vi "Enter_Temp_Press.vi"() -> ()   [LabVIEW 2020]
uses:
  Sub VIs/ADAM Controls/Channel_names.ctl
  Anemometry/Anemometry Sub Vis/Globals/Preference_global.vi
  Anemometry/Anemometry Sub Vis/Globals/Constants_global.vi
  Sub VIs/ADAM Controls/Module_type_ADAM.ctl
  Anemometry/Anemometry Sub Vis/Controls/Preference_Mode.ctl
  Anemometry/Anemometry Sub Vis/File/Setup_Filetype.ctl
  Anemometry/Anemometry Sub Vis/Controls/Server_Comms.ctl
  Sub VIs/ADAM Controls/Update_scan_value.ctl
  <vilib>/Utility/config.llb/NI_LVConfig.lvlib
  <vilib>/Utility/config.llb/Write Key (String).vi
  <vilib>/Utility/config.llb/Write Key (I32).vi
  Sub VIs/ADAM Controls/Function_ADAM.ctl
  Sub VIs/ADAM Controls/Channel_State.ctl
  Sub VIs/ADAM Controls/Calib_type_ADAM.ctl
  Sub VIs/ADAM Controls/Address.ctl
  Sub VIs/ADAM Controls/Ch_description_ADAM.ctl
panel:
  in  "OK":bool
  out "Ch Description Array":T1[](array[typedef]) {"Duty" format="%016b"; "D" format="%#_5g"; "C" format="%#_5g"; "B" format="%#_5g"; "A" format="%#_5g"}
  in  "mbars":dbl format="%#.1f"
  in  "Deg C":dbl format="%#.1f"
  in  "type specifier VI Refnum (for type only)":refnum<vi>
  out "Preference file":path
  in  "Server Comms":T7=enum."Server Link Healthy"
  in  "Browse for Atmos Press":bool
  in  "Browse for Temp Ch":bool
  in  "Flow Pressure (Absolute) (mbars)":string="Froude:NPL:Atmos_Press"
  in  "Flow Temperature (deg C)":string="EnFlo Tun:Inlet Heater:Av Temp"
  # "DATA SOURCE"
  # "CURRENT VALUES"
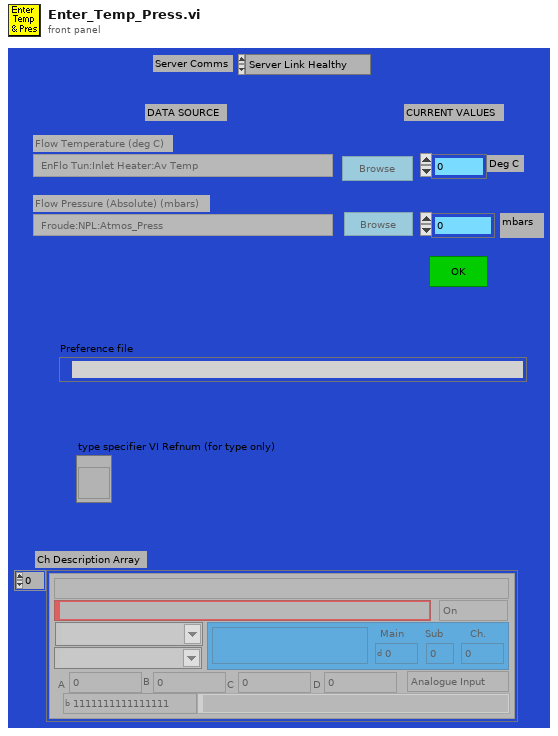
[diagram p1: front panel]
types:
  T1 = typedef "Ch_description_ADAM.ctl" = cluster{"Ch Name":string, "Type":T2, "Function":T3, "Ch State":T4, "Calibration type":T5, "A":dbl, "B":dbl, "C":dbl, "D":dbl, "Comments":string, "Address":T6, "String":string, "Duty":u16}
  T2 = typedef "Module_type_ADAM.ctl" = string
  T3 = typedef "Function_ADAM.ctl" = enum16{"Analogue Input", "Digital Input", "Event counter", "Event rate", "Analogue Output", "Digital Output", "Relay Output"}
  T4 = typedef "Channel_State.ctl" = enum16{"On", "Off", "Always On", "Always Off"}
  T5 = typedef "Calib_type_ADAM.ctl" = string
  T6 = typedef "Address.ctl" = cluster{"Main":i32, "Ch.":i32, "Sub":i32, "Port Name":string}
  T7 = typedef "Server_Comms.ctl" = enum16{"Do Not Link To Server", "Server Link Healthy"}
  T8 = typedef "Setup_Filetype.ctl" = enum16{"Measurement Setups", "Calibration Setups", "General", "Results File Plotter Setups", "Speed Calib Tweaks"}
  T9 = typedef "Channel_names.ctl" = enum16{"Active Only", "Active + Off", "All Channels"}
  T10 = enum16{"Zero or one", "One", "Zero or more", "One or more"}
  T11 = typedef "Preference_Mode.ctl" = enum16{"Load Preferences from file", "Save Preferences to file", "Load, Edit then Save"}
  T12 = typedef "Update_scan_value.ctl" = cluster{"Channel Name":string, "New Value":dbl}
  T13 = typedef "NI_LVConfig.lvlib/Config Data RefNum.ctl" = refnum<k1>
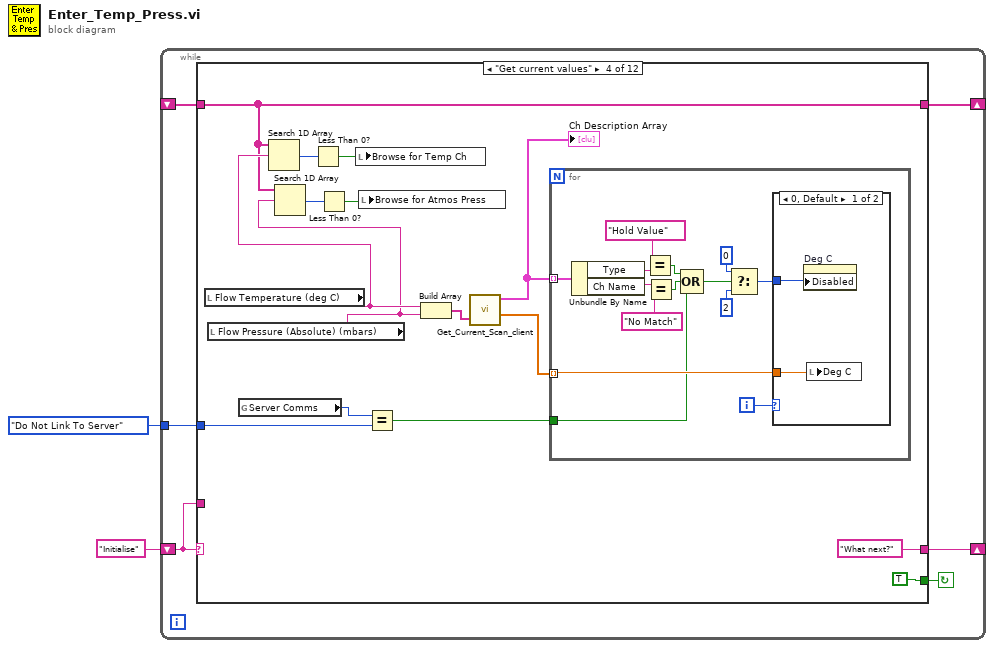
[diagram p0: block diagram]
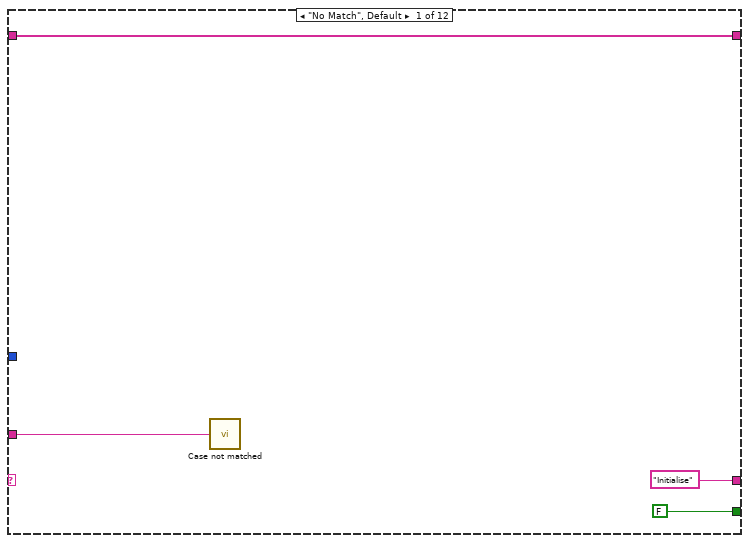
[diagram p2: hidden frame]
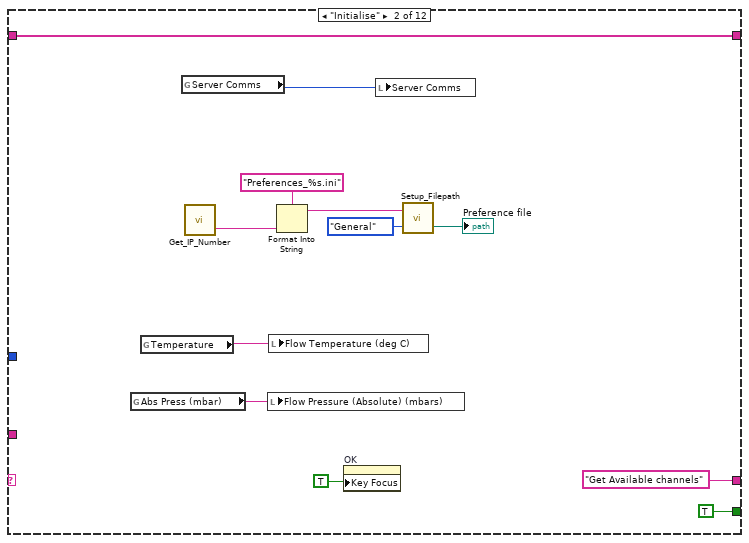
[diagram p3: hidden frame]
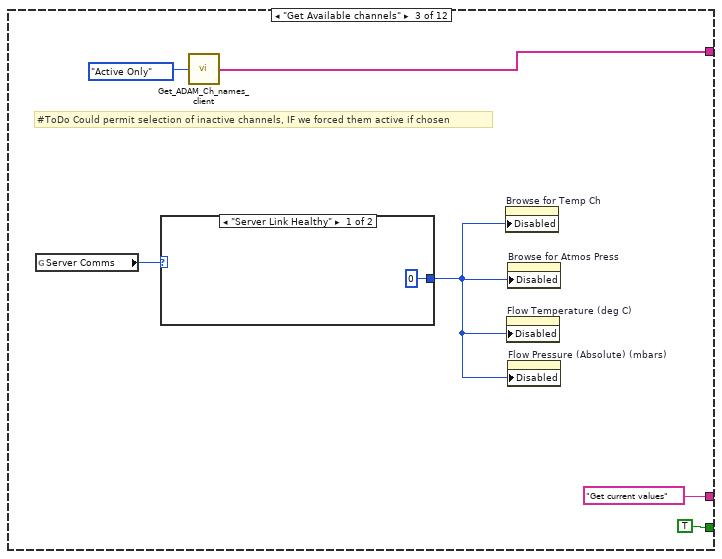
[diagram p4: hidden frame]
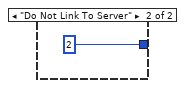
[diagram p5: hidden frame]
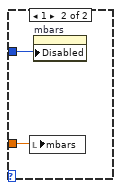
[diagram p6: hidden frame]
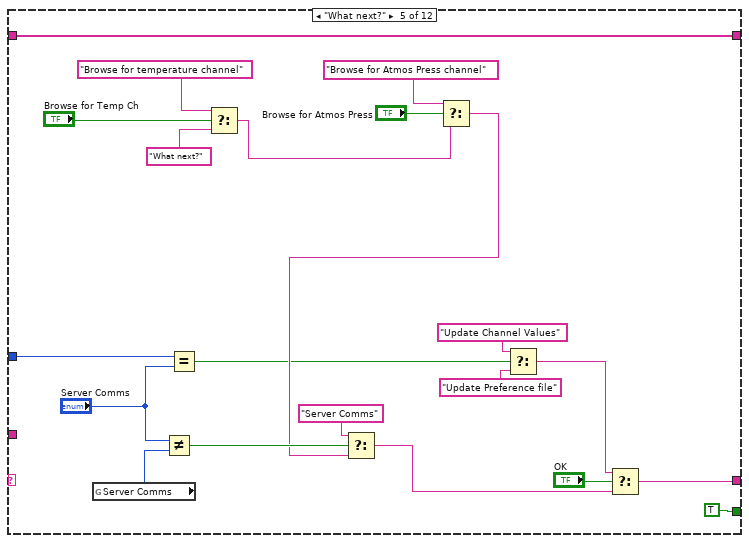
[diagram p7: hidden frame]
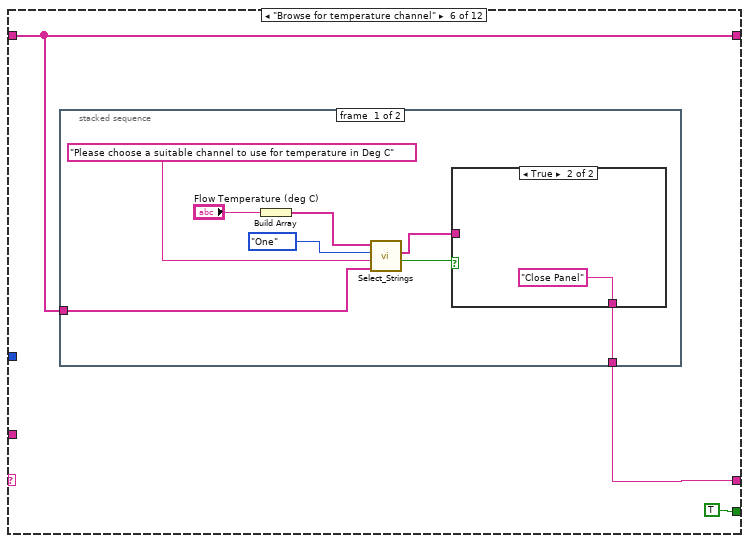
[diagram p8: hidden frame]
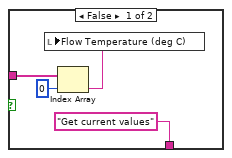
[diagram p9: hidden frame]
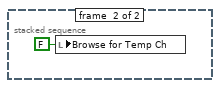
[diagram p10: hidden frame]
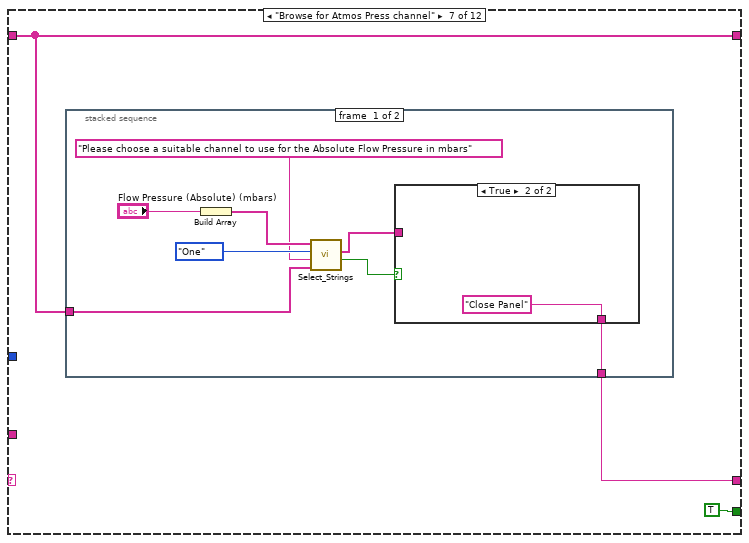
[diagram p11: hidden frame]
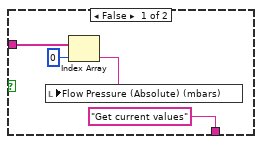
[diagram p12: hidden frame]
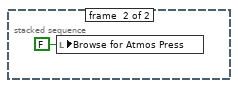
[diagram p13: hidden frame]
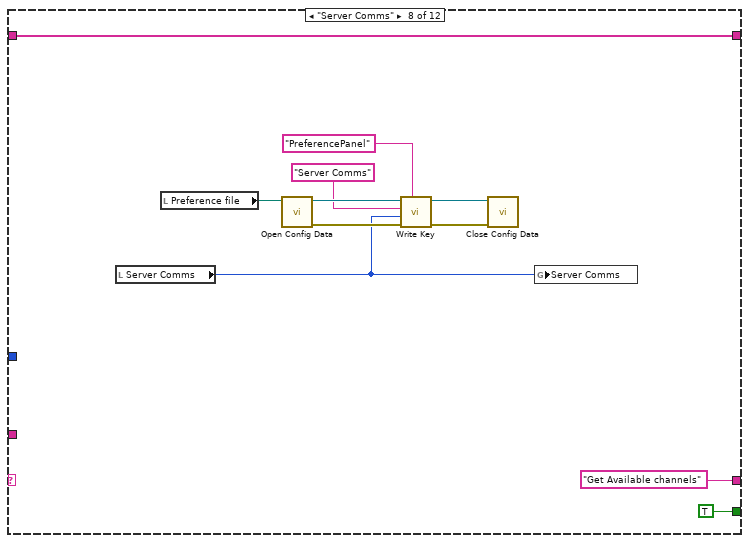
[diagram p14: hidden frame]
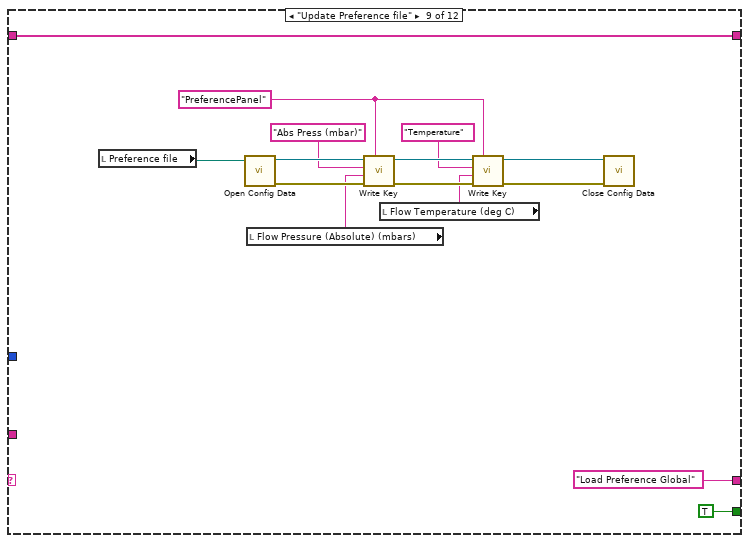
[diagram p15: hidden frame]
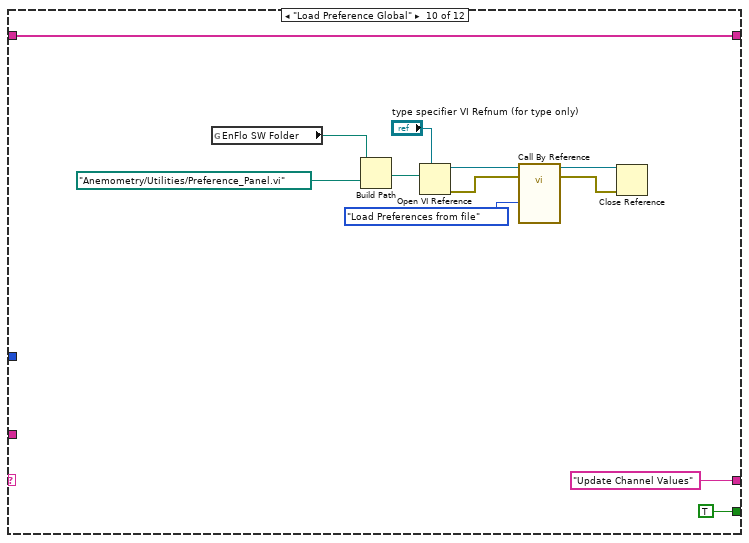
[diagram p16: hidden frame]
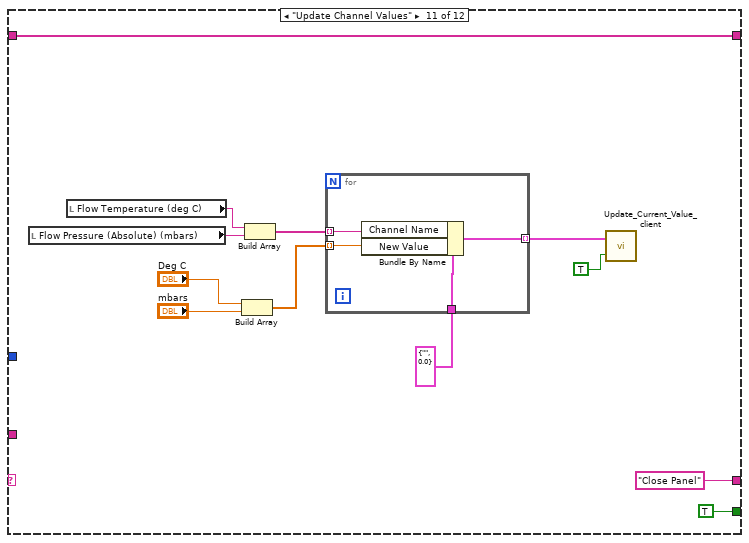
[diagram p17: hidden frame]
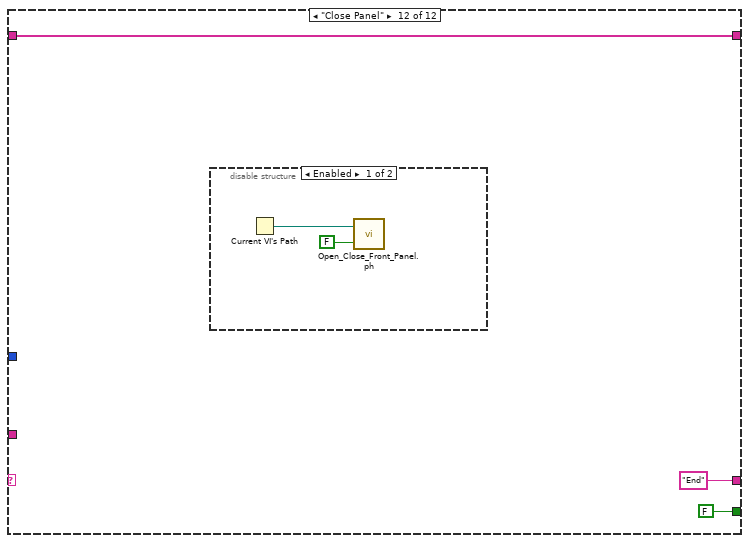
[diagram p18: hidden frame]
diagram:
  n1 = while {
    shift-left: "Initialise" -> [w6]
    shift-right: [w7] -> _
    shift-right: [w5] -> _
    shift-left: _ -> [w4]
    tunnel: Server_Comms."Do Not Link To Server" ("Server Comms") -> [w3]
    stop <- w8 continue-if-true
    n2 = case shown="\"Get current values\"" w6 {
      tunnel: [FALSE TRUE TRUE TRUE TRUE TRUE TRUE TRUE TRUE TRUE TRUE FALSE] -> w8
      tunnel: ["Initialise" "Get Available channels" "Get current values" "What next?" w83 w87 w104 "Get Available channels" "Load Preference Global" "Update Channel Values" "Close Panel" "End"] -> w7
      tunnel: w6 -> [w9 _ _ _ _ _ _ _ _ _ _ _]
      tunnel: [w10 w23 w27 w37 w81 w88 w105 w129 w144 w156 w168 w175] -> w5
      tunnel: w4 -> [w10 w23 _ w37 w81 w88 w105 w129 w144 w156 w168 w175]
      tunnel: w3 -> [_ _ _ w33 w70 _ _ _ _ _ _ _]
      frame "No Match", Default {
        n3 = call "Case not matched.vi"("Case Name not Matched"=w9) -> ()
      }
      frame "Initialise" {
        n4 = global read "Preference_global.vi" "Abs Press (mbar)"() -> (w20:string)
        n5 = global read "Preference_global.vi" "Temperature"() -> (w19:string)
        n6 = global read "Preference_global.vi" "Server Comms"() -> (w24:T7)
        n7 = call "Get_IP_Number.vi"() -> ("bestAvailableName"=w14:string)  [unwired: 1 out]
        n8 = local write "Flow Pressure (Absolute) (mbars)"(w20) -> ()
        n9 = local write "Flow Temperature (deg C)"(w19) -> ()
        n10 = Format Into String(format string="Preferences_%s.ini" ("name or relative path"), w14) -> (resulting string=w13:string)  [unwired: 2 in, 1 out]
        n11 = property on="OK" class="Bool"("Key Focus"=TRUE) -> ()  [unwired: 2 in, 2 out]
        n12 = local write "Server Comms"(w24) -> ()
        n13 = call "Setup_Filepath.vi"("Setup File Type"=Setup_Filetype."General", "Filename in"=w13) -> ("Filename Out"=→"Preference file":path)  [unwired: 1 out]
      }
      frame "Get Available channels" {
        # "#ToDo Could permit selection of inactive channels, IF we forced them active if chosen"
        n14 = global read "Preference_global.vi" "Server Comms"() -> (w26:T7)
        n15 = case shown="\"Server Link Healthy\"" w26 {
          tunnel: [u8 0 ("Disabled") u8 2 ("Disabled")] -> w25
          frame "Server Link Healthy" {
          }
          frame "Do Not Link To Server" {
          }
        }
        n16 = call "Get_ADAM_Ch_names_client.vi"("Channel names set"=Channel_names."Active Only") -> ("Ch names"=w27:string[])
        n17 = property on="Browse for Temp Ch" class="Bool (strict)"("Disabled"=w25) -> ()  [unwired: 2 in, 2 out]
        n18 = property on="Flow Temperature (deg C)" class="Str"("Disabled"=w25) -> ()  [unwired: 2 in, 2 out]
        n19 = property on="Browse for Atmos Press" class="Bool (strict)"("Disabled"=w25) -> ()  [unwired: 2 in, 2 out]
        n20 = property on="Flow Pressure (Absolute) (mbars)" class="Str"("Disabled"=w25) -> ()  [unwired: 2 in, 2 out]
      }
      frame "Get current values" {
        n21 = local read "Flow Temperature (deg C)"() -> (w42:string)
        n22 = local read "Flow Pressure (Absolute) (mbars)"() -> (w36:string)
        n23 = global read "Preference_global.vi" "Server Comms"() -> (w35:T7)
        n24 = Search 1D Array(1D array=w37, element=w42) -> (index of element=w41:i32)  [unwired: 1 out]
        n25 = Search 1D Array(1D array=w37, element=w36) -> (index of element=w40:i32)  [unwired: 1 out]
        n26 = Less Than 0?(x=w41) -> (x < 0?=w39:bool)
        n27 = Less Than 0?(x=w40) -> (x < 0?=w38:bool)
        n28 = local write "Browse for Temp Ch"(w39) -> ()
        n29 = local write "Browse for Atmos Press"(w38) -> ()
        n30 = Equal?(x=w35, y=w33) -> (x = y?=w34:bool)
        n31 = Build Array(w42, w36) -> (w45:string[])
        n32 = call "Get_Current_Scan_client.vi"("multipleChannels"=w45) -> ("Ch Description Array"=w43:T1[], "Numerical Values"=w44:dbl[])  [unwired: 2 in, 1 out]
        "Ch Description Array" <- w43
        n33 = for {
          tunnel: w44 -> [w49] mode=indexing
          tunnel: w43 -> [w60] mode=indexing
          tunnel: w34 -> [w48]
          i -> [w61]
          n34 = Unbundle By Name(w60) -> ("Type"=w59:T2, "Ch Name"=w54:string)
          n35 = Equal?(x=T2 "Hold Value" ("Type"), y=w59) -> (x = y?=w51:bool)
          n36 = Equal?(x=w54, y="No Match") -> (x = y?=w52:bool)
          n37 = Compound Arithmetic op=OR(w51, w52, w48) -> (w50:bool)
          n38 = Select(t=u8 0 ("Disabled"), s=w50, f=u8 2 ("Disabled")) -> (s? t:f=w55:u8)
          n39 = case shown="0, Default" w61 {
            tunnel: w49 -> [w63 w65]
            tunnel: w55 -> [w62 w64]
            frame 0, Default {
              n40 = property on="Deg C" class="DigNum (strict)"("Disabled"=w62) -> ()  [unwired: 2 in, 2 out]
              n41 = local write "Deg C"(w63) -> ()
            }
            frame 1 {
              n42 = local write "mbars"(w65) -> ()
              n43 = property on="mbars" class="DigNum (strict)"("Disabled"=w64) -> ()  [unwired: 2 in, 2 out]
            }
          }
        }
      }
      frame "What next?" {
        n44 = global read "Preference_global.vi" "Server Comms"() -> (w75:T7)
        n45 = Not Equal?(x="Server Comms", y=w75) -> (x != y?=w74:bool)
        n46 = Equal?(x=w70, y="Server Comms") -> (x = y?=w69:bool)
        n47 = Select(t="Browse for temperature channel", s="Browse for Temp Ch", f="What next?") -> (s? t:f=w78:string)
        n48 = Select(t="Browse for Atmos Press channel", s="Browse for Atmos Press", f=w78) -> (s? t:f=w72:string)
        n49 = Select(t="Server Comms", s=w74, f=w72) -> (s? t:f=w77:string)
        n50 = Select(t="Update Channel Values", s=w69, f="Update Preference file") -> (s? t:f=w67:string)
        n51 = Select(t=w67, s="OK", f=w77) -> (s? t:f=w83:string)
      }
      frame "Browse for temperature channel" {
        n52 = stacked-sequence {
          tunnel: w88 -> [w95 _]
          tunnel: [w90 _] -> w87
          frame #0 {
            n53 = Build Array("Flow Temperature (deg C)") -> (w97:string[])
            n54 = call "Select_Strings.vi"("Available Ch names"=w95, "Message"="Please choose a suitable channel to use for temperature in Deg C", "Selector mode"=T10."One", "Desired Ch names (in)"=w97) -> ("Cancel"=w91:bool, "Selected Channel Names"=w94:string[])  [unwired: 1 in, 2 out]
            n55 = case shown="True" w91 {
              tunnel: w94 -> [w101 _]
              tunnel: ["Get current values" "Close Panel"] -> w90
              frame False {
                n56 = Index Array(array=w101, index=0) -> (element=w99:string)
                n57 = local write "Flow Temperature (deg C)"(w99) -> ()
              }
              frame True {
              }
            }
          }
          frame #1 {
            n58 = local write "Browse for Temp Ch"(FALSE ("Browse for Temp Ch")) -> ()
          }
        }
      }
      frame "Browse for Atmos Press channel" {
        n59 = stacked-sequence {
          tunnel: w105 -> [w112 _]
          tunnel: [w107 _] -> w104
          frame #0 {
            n60 = Build Array("Flow Pressure (Absolute) (mbars)") -> (w114:string[])
            n61 = call "Select_Strings.vi"("Available Ch names"=w112, "Message"="Please choose a suitable channel to use for the Absolute Flow Pressure in mbars", "Selector mode"=T10."One", "Desired Ch names (in)"=w114) -> ("Cancel"=w108:bool, "Selected Channel Names"=w111:string[])  [unwired: 1 in, 2 out]
            n62 = case shown="True" w108 {
              tunnel: w111 -> [w118 _]
              tunnel: ["Get current values" "Close Panel"] -> w107
              frame False {
                n63 = Index Array(array=w118, index=0) -> (element=w116:string)
                n64 = local write "Flow Pressure (Absolute) (mbars)"(w116) -> ()
              }
              frame True {
              }
            }
          }
          frame #1 {
            n65 = local write "Browse for Atmos Press"(FALSE ("Browse for Atmos Press")) -> ()
          }
        }
      }
      frame "Server Comms" {
        n66 = local read "Server Comms"() -> (w121:T7)
        n67 = local read "Preference file"() -> (w123:path)
        n68 = call <vilib>:"Open Config Data.vi"("configuration file path"=w123) -> ("error out"=w126:errorcluster, "refnum"=w128:T13)  [unwired: 8 in, 1 out]
        n69 = call-poly <vilib>:"Write Key.vi"("section"="PreferencePanel", "error in (no error)"=w126, "value"=w121, "key"="Server Comms", "refnum"=w128) -> ("error out"=w125:errorcluster, "refnum out"=w127:T13)  [unwired: 4 in, 1 out]
        n70 = call <vilib>:"Close Config Data.vi"("error in (no error)"=w125, "refnum"=w127) -> ()  [unwired: 8 in, 2 out]
        n71 = global write "Preference_global.vi" "Server Comms"(w121) -> ()
      }
      frame "Update Preference file" {
        w132 = "PreferencePanel" ("section")
        n72 = local read "Preference file"() -> (w140:path)
        n73 = call <vilib>:"Open Config Data.vi"("configuration file path"=w140) -> ("error out"=w139:errorcluster, "refnum"=w143:T13)  [unwired: 8 in, 1 out]
        n74 = local read "Flow Pressure (Absolute) (mbars)"() -> (w135:string)
        n75 = call-poly <vilib>:"Write Key.vi"("section"=w132, "error in (no error)"=w139, "value"=w135, "key"="Abs Press (mbar)", "refnum"=w143) -> ("error out"=w138:errorcluster, "refnum out"=w142:T13)  [unwired: 4 in, 1 out]
        n76 = local read "Flow Temperature (deg C)"() -> (w133:string)
        n77 = call-poly <vilib>:"Write Key.vi"("section"=w132, "error in (no error)"=w138, "value"=w133, "key"="Temperature", "refnum"=w142) -> ("error out"=w137:errorcluster, "refnum out"=w141:T13)  [unwired: 4 in, 1 out]
        n78 = call <vilib>:"Close Config Data.vi"("error in (no error)"=w137, "refnum"=w141) -> ()  [unwired: 8 in, 2 out]
      }
      frame "Load Preference Global" {
        n79 = global read "Constants_global.vi" "EnFlo SW Folder"() -> (w149:path)
        n80 = Build Path(base path=w149, name or relative path=path "Anemometry/Utilities/Preference_Panel.vi") -> (appended path=w151:path)
        n81 = Open VI Reference(type specifier VI Refnum (for type only)="type specifier VI Refnum (for type only)", vi path=w151) -> (vi reference=w152:refnum<vi>, error out=w153:errorcluster)  [unwired: 1 in, 3 out]
        n82 = call-by-ref "?"(reference=w152, error in=w153, "Mode"=Preference_Mode."Load Preferences from file") -> (reference out=w154:refnum<vi>, error out=w155:errorcluster)
        n83 = Close Reference(reference=w154, error in (no error)=w155) -> ()  [unwired: 1 out]
      }
      frame "Update Channel Values" {
        n84 = local read "Flow Pressure (Absolute) (mbars)"() -> (w165:string)
        n85 = local read "Flow Temperature (deg C)"() -> (w164:string)
        n86 = Build Array("Deg C", "mbars") -> (w162:dbl[])
        n87 = Build Array(w164, w165) -> (w163:string[])
        n88 = for {
          tunnel: w163 -> [w174] mode=indexing
          tunnel: w162 -> [w173] mode=indexing
          tunnel: T12 {"Channel Name"="", "New Value"=0.0} ("Update Scan Value Cluster") -> [w172]
          tunnel: [w171] -> w160 mode=indexing
          n89 = Bundle By Name(cluster=w172, "Channel Name"=w174, "New Value"=w173) -> (w171:T12)
        }
        n90 = call "Update_Current_Value_client.vi"("Don't Bother with check?"=TRUE, "Update array in"=w160) -> ()
      }
      frame "Close Panel" {
        n91 = disable-structure shown="Enabled" {
          frame Enabled {
            n92 = Current VI's Path() -> (path=w179:path)
            n93 = call "Open_Close_Front_Panel.ph.vi"("Front Panel Window:Open"=FALSE, "VI path"=w179) -> ()  [unwired: 2 out]
          }
          frame Disabled {
          }
        }
      }
    }
  }
